vi "gxml_XMLArraySizes.vi"(7 "NDims":i32, 8 "error in":errorcluster, 11 "Item Data":T1) -> (0 "error out":errorcluster, 2 "XML Array Empty?":bool, 3 "Dim Sizes":i32[](array[numeric]))   [LabVIEW 2011, in "Third Party VIs.lvlib" / "GXML.lvlib"]
uses:
  <vilib>/regexp/Match Regular Expression.xnode
  GXML.lvlib
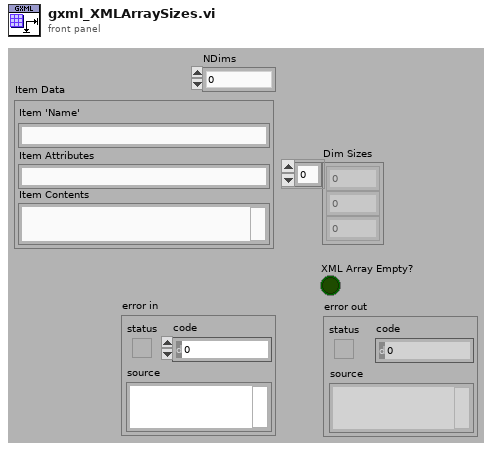
[diagram p1: front panel]
types:
  T1 = cluster{"Item 'Name'":string, "Item Attributes":string, "Item Contents":string}
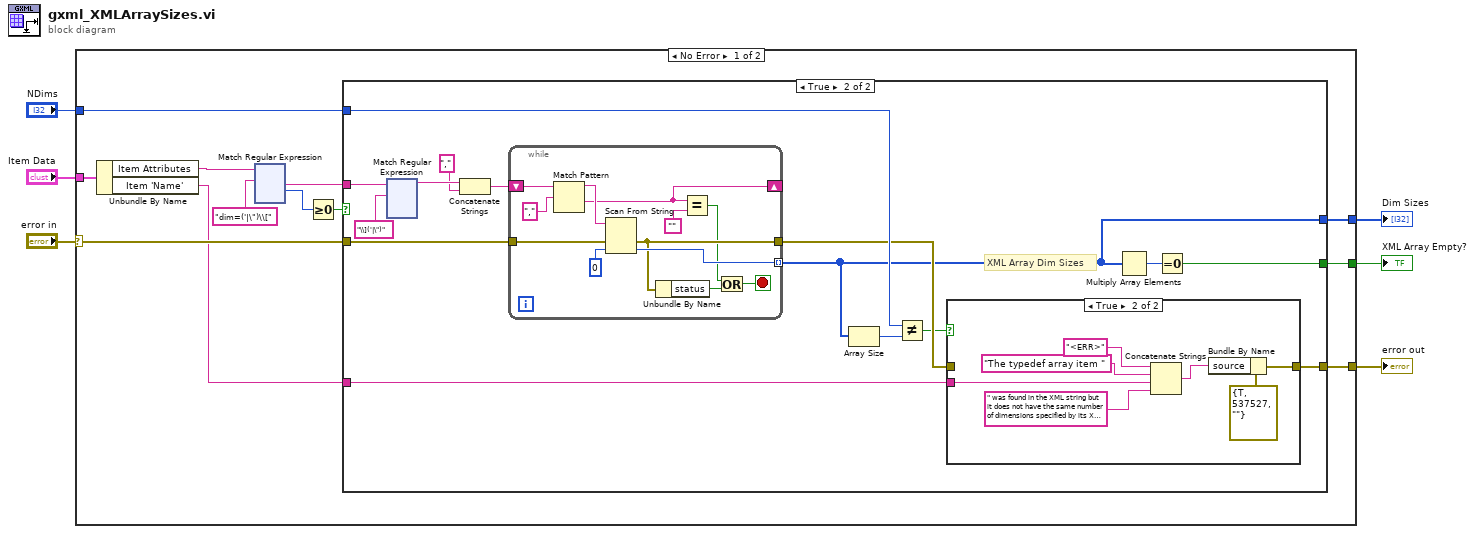
[diagram p0: block diagram]
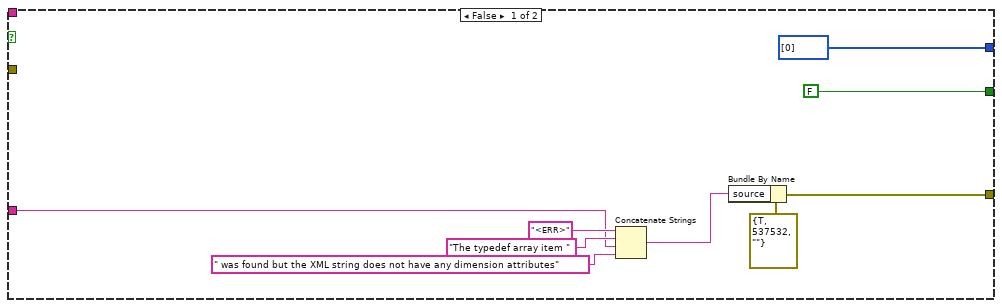
[diagram p2: hidden frame]
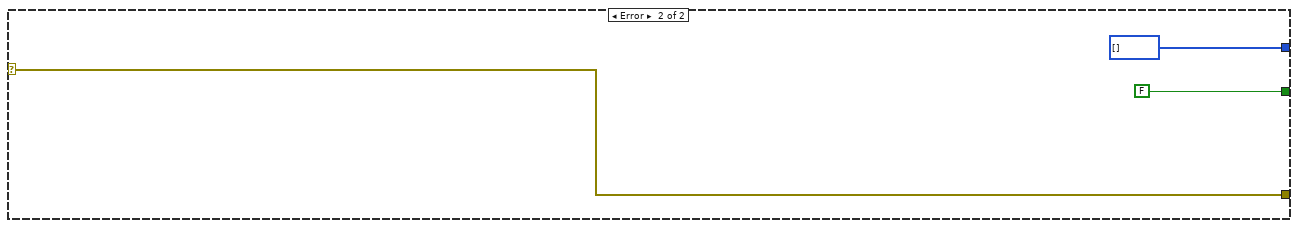
[diagram p4: hidden frame]
diagram:
  n1 = case shown="No Error" "error in" {
    selector: "error in" -> [w10 w287]
    tunnel: "NDims" -> [w18 _]
    tunnel: [w17 w287] -> w5
    tunnel: "Item Data" -> [w16 _]
    tunnel: [w15 i32[] []] -> w3
    tunnel: [w14 FALSE] -> w2
    frame No Error {
      n2 = Unbundle By Name(w16) -> ("Item Attributes"=w9:string, "Item 'Name'"=w7:string)
      n3 = xnode "Match Regular Expression"("input string"=w9, "regular expression"="dim=('|\")\\[") -> ("after match"=w12:string, "offset past match"=w8:i32)  [unwired: 4 in, 3 out]
      n4 = Greater Or Equal To 0?(x=w8) -> (x >= 0?=w11:bool)
      n5 = case shown="True" w11 {
        tunnel: w18 -> [_ w153]
        tunnel: [w131 w152] -> w17
        tunnel: w10 -> [_ w148]
        tunnel: [i32[] [0] w147] -> w15
        tunnel: [FALSE w146] -> w14
        tunnel: w12 -> [_ w140]
        tunnel: w7 -> [w130 w139]
        frame False {
          n6 = Concatenate Strings("<ERR>" ("source"), "The typedef array item " ("string"), w130, " was found but the XML string does not have any dimension attributes" ("string")) -> (w135:string)
          n7 = Bundle By Name(cluster=errorcluster {"status"=TRUE, "code"=537532, "source"=""} ("error in"), "source"=w135) -> (w131:errorcluster)
        }
        frame True {
          # "XML Array Dim Sizes"
          n8 = xnode "Match Regular Expression"("input string"=w140, "regular expression"="\\]('|\")") -> ("before match"=w143:string)  [unwired: 4 in, 4 out]
          n9 = Concatenate Strings(w143, ",") -> (w141:string)
          n10 = while {
            shift-right: [w272] -> _
            shift-left: w141 -> [w274]
            tunnel: [w271] -> w147 mode=indexing
            tunnel: w148 -> [w270]
            tunnel: [w268] -> w151
            stop <- w265 stop-if-true
            n11 = Match Pattern(string=w274, regular expression=",") -> (before substring=w273:string, after substring=w272:string)  [unwired: 1 in, 2 out]
            n12 = Scan From String(input string=w273, error in=w270, default 1=0) -> (error out=w268:errorcluster, output 1=w271:i32)  [unwired: 2 in, 2 out]
            n13 = Unbundle By Name(w268) -> ("status"=w267:bool)
            n14 = Equal?(x=w272, y="") -> (x = y?=w266:bool)
            n15 = Or(x=w266, y=w267) -> (x .or. y?=w265:bool)
          }
          n16 = Array Size(array=w147) -> (size(s)=w145:i32)
          n17 = Not Equal?(x=w153, y=w145) -> (x != y?=w150:bool)
          n18 = case shown="True" w150 {
            tunnel: w151 -> [w277 _]
            tunnel: [w277 w284] -> w152
            tunnel: w139 -> [_ w278]
            frame False {
            }
            frame True {
              n19 = Concatenate Strings("<ERR>" ("source"), "The typedef array item " ("string"), w278, " was found in the XML string but it does not have the same number of dimensions specified by its XML attribute." ("string")) -> (w279:string)
              n20 = Bundle By Name(cluster=errorcluster {"status"=TRUE, "code"=537527, "source"=""} ("error in"), "source"=w279) -> (w284:errorcluster)
            }
          }
          n21 = Multiply Array Elements(1:w147) -> (0:w149:i32)
          n22 = Equal To 0?(x=w149) -> (x = 0?=w146:bool)
        }
      }
    }
    frame Error {
    }
  }
  "Dim Sizes" <- w3
  "error out" <- w5
  "XML Array Empty?" <- w2
